vi "Store Waveform to Reference Channel.vi"(6 "Waveform File":string, 8 "error in (no error)":errorcluster, 9 "Reference Channel (5: Reference 1)":u16(ring)=5 items=["Reference 1"=5, "Reference 2"=6, "Reference 3"=7, "Reference 4"=8, "Edit Memory"=25, "Arbitrary Memory 1"=26, "Arbitrary Memory 2"=27, "Arbitrary Memory 3"=28, "Arbitrary Memory 4"=29, "Waveform File"=50], 10 "Source Channel (0: Channel 1)":u16(ring) items=["Channel 1", "Channel 2", "Channel 3", "Channel 4", "Math", "Reference 1", "Reference 2", "Reference 3", "Reference 4", "Digital Channel 0", "Digital Channel 1", "Digital Channel 2", "Digital Channel 3", "Digital Channel 4", "Digital Channel 5", "Digital Channel 6", "Digital Channel 7", "Digital Channel 8", "Digital Channel 9", "Digital Channel 10", "Digital Channel 11", "Digital Channel 12", "Digital Channel 13", "Digital Channel 14", "Digital Channel 15", "Edit Memory", "Arbitrary Memory 1", "Arbitrary Memory 2", "Arbitrary Memory 3", "Arbitrary Memory 4", "Normal", "Average", "Maximum Peak Hold", "Minimum Peak Hold", "Baseband I & Q Data", "All"], 11 "VISA resource name":refnum<visa-resource-name>) -> (0 "error out":errorcluster, 3 "VISA resource name out":refnum<visa-resource-name>)   [LabVIEW 2016, in "Tektronix DPO MSO 2000 4000 Series.lvlib"]
doc: "Stores a waveform to a reference channel."
uses:
  Tektronix DPO MSO 2000 4000 Series.lvlib
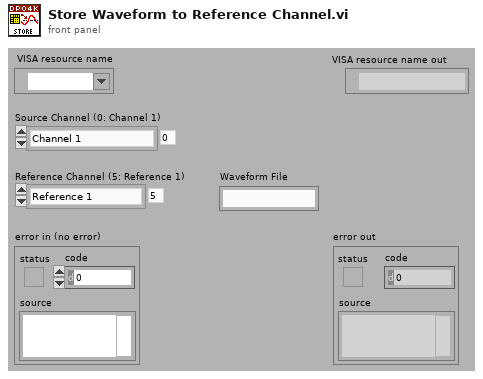
[diagram p1: front panel]
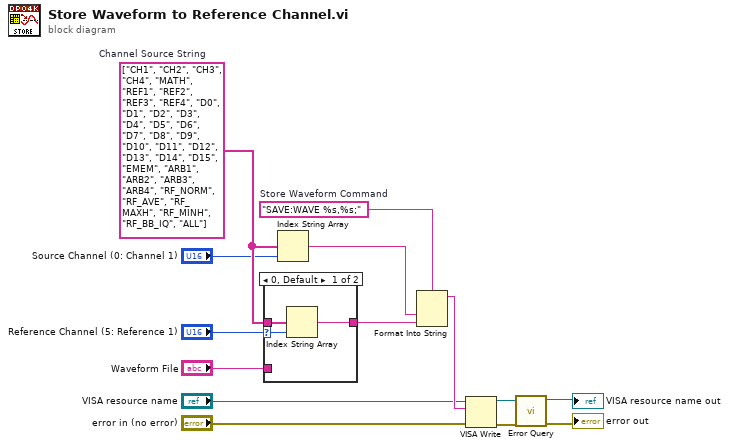
[diagram p0: block diagram]
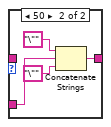
[diagram p2: hidden frame]
diagram:
  w14 = "SAVE:WAVE %s,%s;"  # Store Waveform Command
  w9 = string[] ["CH1", "CH2", "CH3", "CH4", "MATH", "REF1", "REF2", "REF3", "REF4", "D0", "D1", "D2", "D3", "D4", "D5", "D6", "D7", "D8", "D9", "D10", "D11", "D12", "D13", "D14", "D15", "EMEM", "ARB1", "ARB2", "ARB3", "ARB4", "RF_NORM", "RF_AVE", "RF_MAXH", "RF_MINH", "RF_BB_IQ", "ALL"]  # Channel Source String
  n1 = case shown="0, Default" "Reference Channel (5: Reference 1)" {
    selector: "Reference Channel (5: Reference 1)" -> [w15 _]
    tunnel: [w17 w21] -> w12
    tunnel: w9 -> [w16 _]
    tunnel: "Waveform File" -> [_ w20]
    frame 0, Default {
      n2 = Index String Array(1:w15, 2:w16) -> (0:w17:string)  [unwired: 1 in]
    }
    frame 50 {
      n3 = Concatenate Strings("\"" ("string"), w20, "\"" ("string")) -> (w21:string)
    }
  }
  n4 = Index String Array(1:"Source Channel (0: Channel 1)", 2:w9) -> (0:w13:string)  [unwired: 1 in]
  n5 = Format Into String(format string=w14, w13, w12) -> (resulting string=w7:string)  [unwired: 2 in, 1 out]
  n6 = VISA Write(VISA resource name="VISA resource name", write buffer=w7, error in (no error)="error in (no error)") -> (VISA resource name out=w4:refnum<visa-resource-name>, error out=w3:errorcluster)  [unwired: 1 out]
  n7 = call "Error Query.vi"("error in (no error)"=w3, "VISA resource name"=w4) -> ("error out"=→"error out":errorcluster, "VISA resource name out"=→"VISA resource name out":refnum<visa-resource-name>)  [unwired: 6 in, 2 out]
